vi "run.vi"(8 "error in (no error)":errorcluster, 11 "DAQ_DL090211Scaffold in":refnum<class "DAQ_DL090211Scaffold.lvclass">) -> (0 "error out":errorcluster, 3 "DAQ_DL090211Scaffold out":refnum<class "DAQ_DL090211Scaffold.lvclass">)   [LabVIEW 2010, in "DAQ_DL090211Scaffold.lvclass"]
uses:
  DAQ_DL090211Scaffold.lvclass
  internal_trigger_enum.ctl
  state_enum.ctl
  GenericDAQ/GenericDAQ/GenericDAQ.lvclass
  GenericDAQ/GenericDAQ/trigger_enum.ctl
  common/classes/ErrorController/ErrorController/class_data.vi
  common/classes/ErrorController/ErrorController/ErrorController.lvclass
panel:
  in  "Tab Control":enum32{"User", "Debug", "About"}(tab)
  out "terminate?":bool
  out "statechart loop counter":i32
  out "statechart error":errorcluster
  out "last trigger":T1
  out "loop time":u32
  # "This component has no user interface."
  # "DAQ_DL090211Scaffold\n\nImplemented by:\n- Dominik Langer, University of Zurich, Switzerland"
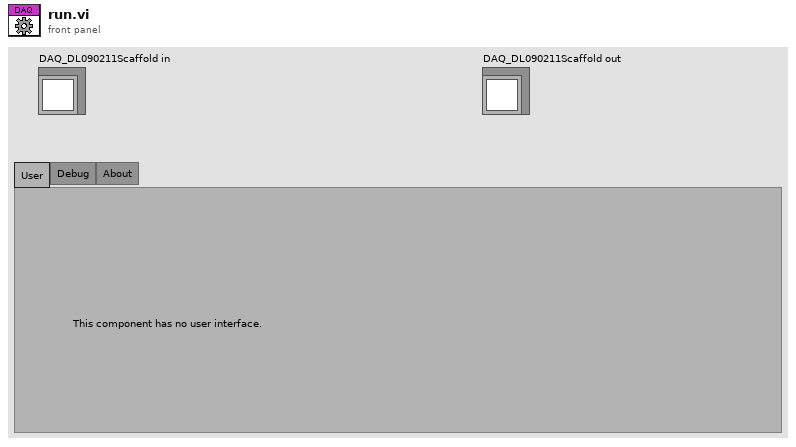
[diagram p1: front panel]
types:
  T1 = typedef "DAQ_DL090211Scaffold.lvclass/internal_trigger_enum.ctl" = enum16{"NULL", "initialise", "terminate", "start", "stop", "read", "attach observer", "detach observer", "reset"}
  T2 = typedef "DAQ_DL090211Scaffold.lvclass/state_enum.ctl" = enum16{"not acquiring", "acquiring"}
  T3 = typedef "GenericDAQ.lvclass/trigger_enum.ctl" = enum16{"NULL", "read"}
  T4 = typedef "top-level_component_type_enum.ctl" = enum16{"undefined", "ImagingMode", "ScanHead", "DAQ", "ImageAssembler", "Display", "DataCollection", "Analyser", "Stimulator", "ExperimentController", "Instrument", "Stage"}
  T5 = typedef "main_trigger_enum.ctl" = enum16{"NULL", "initialise", "terminate", "start", "stop", "change objective", "change experimentController", "change imagingMode", "save notebook", "started saving", "finished saving", "expCtr ready", "expCtr missing", "imgMd ready", "imgMd missing", "scanHd ready", "scanHd missing", "DAQ ready", "DAQ missing", "imgAsm ready", "imgAsm missing", "dataColl ready", "dataColl missing", "display ready", "display missing", "analysr ready", "analysr missing", "instrmnt ready", "instrmnt missing", "stimltr ready", "stimltr missing", "stage ready", "stage missing"}
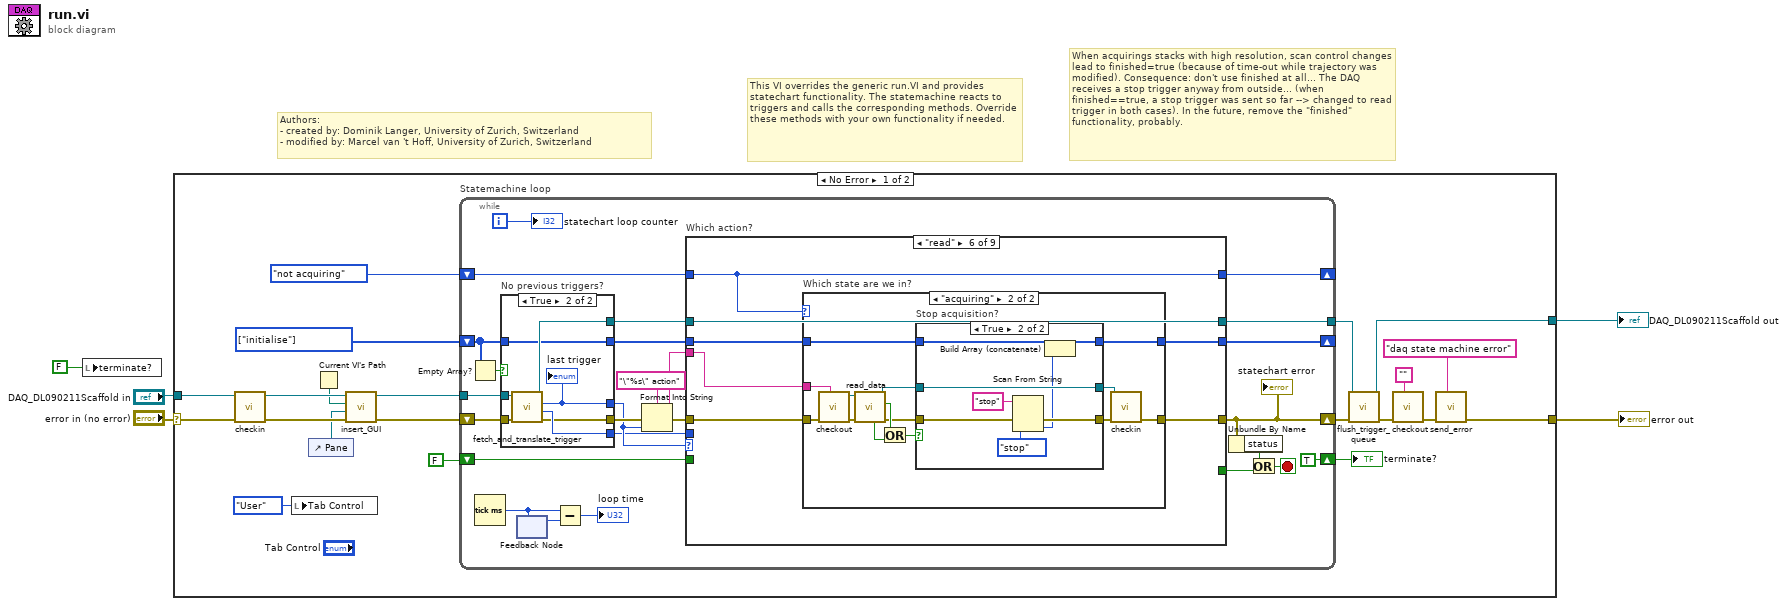
[diagram p0: block diagram]
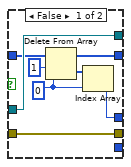
[diagram p2: hidden frame]
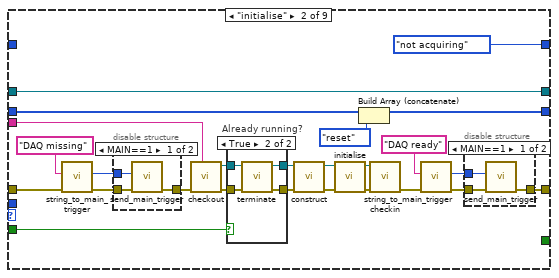
[diagram p4: hidden frame]
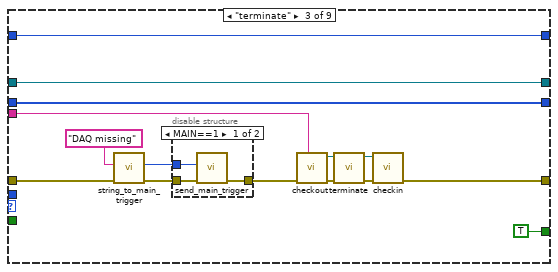
[diagram p8: hidden frame]
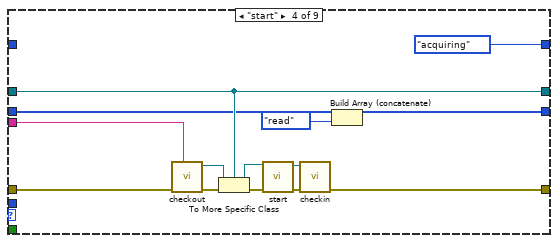
[diagram p10: hidden frame]
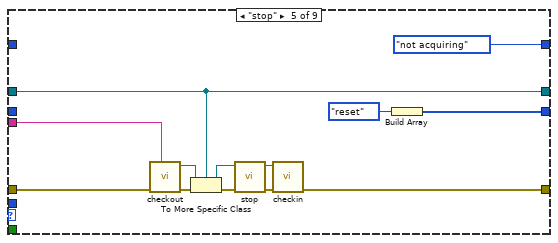
[diagram p11: hidden frame]
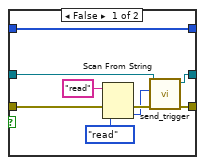
[diagram p13: hidden frame]
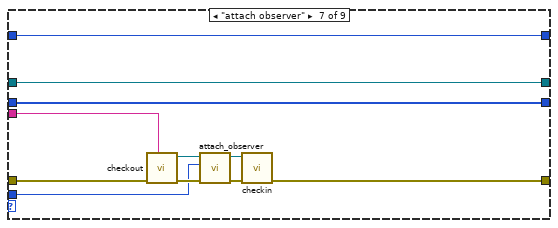
[diagram p14: hidden frame]
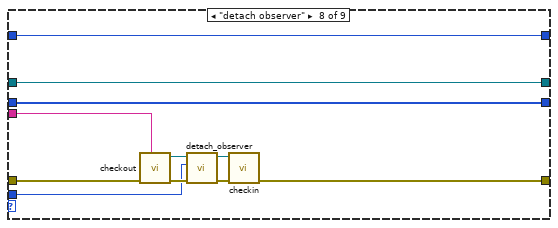
[diagram p15: hidden frame]
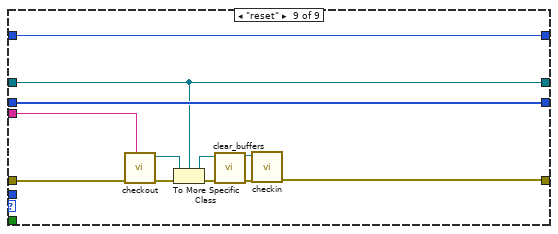
[diagram p16: hidden frame]
diagram:
  # "When acquirings stacks with high resolution, scan control changes lead to finished=true (because of time-out while trajectory was modified). Consequence: don't use finished at all... The DAQ receives a stop trigger anyway from outside... (when finished==true, a stop trigger was sent so far --> changed to read trigger in both cases). In the future, remove the \"finished\" functionality, probably."
  # "This VI overrides the generic run.VI and provides statechart functionality. The statemachine reacts to triggers and calls the corresponding methods. Override these methods with your own functionality if needed."
  # "Authors: \n- created by: Dominik Langer, University of Zurich, Switzerland\n- modified by: Marcel van 't Hoff, University of Zurich, Switzerland"
  n1 = local write "terminate?"(FALSE ("read data?")) -> ()
  n2 = case shown="No Error" "error in (no error)" {
    selector: "error in (no error)" -> [w15 w232]
    tunnel: [w6 w232] -> w4
    tunnel: [w17 w231] -> w2
    tunnel: "DAQ_DL090211Scaffold in" -> [w16 w231]
    frame No Error {
      w14 = T1[] [enum."initialise"] items=["NULL", "initialise", "terminate", "start", "stop", "read", "attach observer", "detach observer", "reset"]
      n3 = call-dynamic "checkin.vi"("error in (no error)"=w15, "GenericDAQ in"=w16) -> ("error out"=w21:errorcluster, "GenericDAQ out"=w23:refnum<class "DAQ_DL090211Scaffold.lvclass">)  [unwired: 8 in]
      n4 = local write "Tab Control"(enum32{"User", "Debug", "About"}."User" ("Tab Control")) -> ()
      n5 = control-ref of="Pane"() -> (w8:refnum<vi>)
      n6 = Current VI's Path() -> (path=w9:path)
      n7 = call-dynamic "insert_GUI.vi"("error in (no error)"=w21, "Pane"=w8, "VI path"=w9, "GenericComponent in"=w23) -> ("error out"=w7:errorcluster, "GenericComponent out"=w12:refnum<class "DAQ_DL090211Scaffold.lvclass">)  [unwired: 6 in]
      n8 = while "Statemachine loop" {
        shift-right: [TRUE] -> w11
        shift-left: FALSE -> [w45]
        shift-right: [w44] -> w20
        shift-left: w7 -> [w48]
        tunnel: w12 -> [w49]
        tunnel: [w46] -> w18
        shift-right: [w40] -> _
        shift-left: w14 -> [w39]
        shift-right: [w32] -> _
        shift-left: state_enum."not acquiring" ("state") -> [w33]
        i -> [w51]
        stop <- w50 stop-if-true
        n9 = Empty Array?(array=w39) -> (empty?=w38:bool)
        n10 = Tick Count (ms)() -> (millisecond timer value=w29:u32)
        n11 = case "No previous triggers?" shown="True" w38 {
          tunnel: w49 -> [w60 w67]
          tunnel: w48 -> [w58 w66]
          tunnel: [w60 w65] -> w47
          tunnel: [w56 w64] -> w31
          tunnel: [_ w63] -> w30
          tunnel: [w58 w62] -> w36
          tunnel: w39 -> [w59 w61]
          tunnel: [w55 w61] -> w41
          frame False {
            w53 = 0 ("index")
            n12 = Delete From Array(array=w59, length=1, index=w53) -> (deleted portion=w57:T1[], array with subset deleted=w55:T1[])
            n13 = Index Array(array=w57, index=w53) -> (element=w56:T1)
          }
          frame True {
            n14 = call-dynamic "fetch_and_translate_trigger.vi"("error in (no error)"=w66, "DAQ_DL090211Scaffold in"=w67) -> ("error out"=w62:errorcluster, "sender TLC type"=w63:T4, "trigger"=w64:T1, "DAQ_DL090211Scaffold out"=w65:refnum<class "DAQ_DL090211Scaffold.lvclass">)  [unwired: 6 in]
            "last trigger" <- w64
          }
        }
        n15 = feedback-in #1(w29) -> ()
        n16 = feedback #1() -> (w28:u32)  [unwired: 1 in]
        n17 = Subtract(x=w29, y=w28) -> (x-y=→"loop time":u32)
        n18 = Format Into String(format string="\"%s\" action", error in=w36, w31) -> (resulting string=w34:string, error out=w37:errorcluster)  [unwired: 1 in]
        n19 = case "Which action?" shown="\"read\"" w31 {
          tunnel: w47 -> [w71 w96 w125 w136 w150 w163 w207 w218 w220]
          tunnel: [w71 w96 w125 w136 w150 w163 w207 w218 w220] -> w46
          tunnel: w30 -> [_ _ _ _ _ _ w201 w212 _]
          tunnel: w37 -> [w70 w79 w114 w137 w149 w162 w202 w213 w223]
          tunnel: [w70 w76 w120 w135 w148 w161 w200 w211 w222] -> w44
          tunnel: w45 -> [_ w87 _ _ _ _ _ _ _]
          tunnel: [_ _ TRUE _ _ _ _ _ _] -> w42
          tunnel: w41 -> [w69 w85 w117 w133 _ w158 w199 w210 w230]
          tunnel: [w69 w84 w117 w132 w145 w157 w199 w210 w230] -> w40
          tunnel: w34 -> [_ w86 w116 w134 w147 w160 w198 w209 w221]
          tunnel: w33 -> [w68 _ w115 _ _ w159 w197 w208 w219]
          tunnel: [w68 state_enum."not acquiring" ("state") w115 state_enum."acquiring" ("state") state_enum."not acquiring" ("state") w159 w197 w208 w219] -> w32
          frame "NULL", Default {
          }
          frame "initialise" {
            n20 = call "string_to_main_trigger.vi"("error in (no error)"=w79, "trigger string"="DAQ missing" ("input string")) -> ("error out"=w78:errorcluster, "main trigger"=w80:T5)  [unwired: 8 in]
            n21 = disable-structure shown="MAIN==1" {
              disable-tunnel: w78 -> [w99 w100]
              disable-tunnel: [w98 w100] -> w81
              disable-tunnel: w80 -> [w97 _]
              frame condition #0 (active) {
                n22 = call "send_main_trigger.vi"("error in (no error)"=w99, "trigger"=w97) -> ("error out"=w98:errorcluster)  [unwired: 9 in]
              }
              frame condition #1 {
              }
            }
            n23 = call "checkout.vi"("locked by?"=w86, "error in (no error)"=w81) -> ("error out"=w92:errorcluster, "GenericDAQ out"=w95:refnum<class "GenericDAQ.lvclass">)  [unwired: 8 out]
            n24 = case "Already running?" shown="True" w87 {
              tunnel: w92 -> [w105 w110]
              tunnel: [w105 w109] -> w93
              tunnel: [w106 w108] -> w94
              tunnel: w95 -> [w106 w107]
              frame False {
              }
              frame True {
                n25 = call-dynamic "terminate.vi"("error in (no error)"=w110, "GenericPlugin in"=w107) -> ("error out"=w109:errorcluster, "GenericPlugin out"=w108:refnum<class "GenericDAQ.lvclass">)  [unwired: 8 out]
              }
            }
            n26 = call-dynamic "construct.vi"("error in (no error)"=w93, "GenericPlugin in"=w94) -> ("error out"=w89:errorcluster, "GenericPlugin out"=w90:refnum<class "GenericDAQ.lvclass">)  [unwired: 2 in, 6 out]
            n27 = call-dynamic "initialise.vi"("error in (no error)"=w89, "GenericPlugin in"=w90) -> ("error out"=w91:errorcluster, "GenericPlugin out"=w88:refnum<class "GenericDAQ.lvclass">)  [unwired: 8 out]
            n28 = Build Array (concatenate)(w85, internal_trigger_enum."reset" ("last trigger 2")) -> (w84:T1[])
            n29 = call-dynamic "checkin.vi"("error in (no error)"=w91, "GenericDAQ in"=w88) -> ("error out"=w75:errorcluster)  [unwired: 8 in, 1 out]
            n30 = call "string_to_main_trigger.vi"("error in (no error)"=w75, "trigger string"="DAQ ready" ("input string")) -> ("error out"=w74:errorcluster, "main trigger"=w72:T5)  [unwired: 8 in]
            n31 = disable-structure shown="MAIN==1" {
              disable-tunnel: w74 -> [w103 w104]
              disable-tunnel: [w102 w104] -> w76
              disable-tunnel: w72 -> [w101 _]
              frame condition #0 (active) {
                n32 = call "send_main_trigger.vi"("error in (no error)"=w103, "trigger"=w101) -> ("error out"=w102:errorcluster)  [unwired: 9 in]
              }
              frame condition #1 {
              }
            }
          }
          frame "terminate" {
            n33 = call "string_to_main_trigger.vi"("error in (no error)"=w114, "trigger string"="DAQ missing" ("input string")) -> ("error out"=w113:errorcluster, "main trigger"=w111:T5)  [unwired: 8 in]
            n34 = disable-structure shown="MAIN==1" {
              disable-tunnel: w113 -> [w128 w129]
              disable-tunnel: [w127 w129] -> w118
              disable-tunnel: w111 -> [w126 _]
              frame condition #0 (active) {
                n35 = call "send_main_trigger.vi"("error in (no error)"=w128, "trigger"=w126) -> ("error out"=w127:errorcluster)  [unwired: 9 in]
              }
              frame condition #1 {
              }
            }
            n36 = call "checkout.vi"("locked by?"=w116, "error in (no error)"=w118) -> ("error out"=w124:errorcluster, "GenericDAQ out"=w123:refnum<class "GenericDAQ.lvclass">)  [unwired: 8 out]
            n37 = call-dynamic "terminate.vi"("error in (no error)"=w124, "GenericPlugin in"=w123) -> ("error out"=w122:errorcluster, "GenericPlugin out"=w121:refnum<class "GenericDAQ.lvclass">)  [unwired: 8 out]
            n38 = call-dynamic "checkin.vi"("error in (no error)"=w122, "GenericDAQ in"=w121) -> ("error out"=w120:errorcluster)  [unwired: 8 in, 1 out]
          }
          frame "start" {
            n39 = call "checkout.vi"("locked by?"=w134, "error in (no error)"=w137) -> ("error out"=w143:errorcluster, "GenericDAQ out"=w142:refnum<class "GenericDAQ.lvclass">)  [unwired: 8 out]
            n40 = To More Specific Class(target class=w136, reference=w142, error in=w143) -> (specific class reference=w140:refnum<class "DAQ_DL090211Scaffold.lvclass">, error out=w141:errorcluster)
            n41 = call-dynamic "start.vi"("error in (no error)"=w141, "DL090211DAQScaffold in"=w140) -> ("error out"=w139:errorcluster, "DL090211DAQScaffold out"=w138:refnum<class "DAQ_DL090211Scaffold.lvclass">)  [unwired: 8 out]
            n42 = call-dynamic "checkin.vi"("error in (no error)"=w139, "GenericDAQ in"=w138) -> ("error out"=w135:errorcluster)  [unwired: 8 in, 1 out]
            n43 = Build Array (concatenate)(w133, internal_trigger_enum."read" ("last trigger 2")) -> (w132:T1[])
          }
          frame "stop" {
            n44 = call "checkout.vi"("locked by?"=w147, "error in (no error)"=w149) -> ("error out"=w156:errorcluster, "GenericDAQ out"=w155:refnum<class "GenericDAQ.lvclass">)  [unwired: 8 out]
            n45 = To More Specific Class(target class=w150, reference=w155, error in=w156) -> (specific class reference=w153:refnum<class "DAQ_DL090211Scaffold.lvclass">, error out=w154:errorcluster)
            n46 = call-dynamic "stop.vi"("error in (no error)"=w154, "DAQ_DL090211Scaffold in"=w153) -> ("error out"=w152:errorcluster, "DAQ_DL090211Scaffold out"=w151:refnum<class "DAQ_DL090211Scaffold.lvclass">)  [unwired: 8 in]
            n47 = call-dynamic "checkin.vi"("error in (no error)"=w152, "GenericDAQ in"=w151) -> ("error out"=w148:errorcluster)  [unwired: 8 in, 1 out]
            n48 = Build Array(internal_trigger_enum."reset" ("last trigger 2")) -> (w145:T1[])
          }
          frame "read" {
            n49 = case "Which state are we in?" shown="\"acquiring\"" w159 {
              tunnel: w162 -> [w165 w179]
              tunnel: [w165 w172] -> w161
              tunnel: w160 -> [_ w169]
              tunnel: w158 -> [w164 w167]
              tunnel: [w164 w166] -> w157
              frame "not acquiring", Default {
              }
              frame "acquiring" {
                n50 = call "checkout.vi"("locked by?"=w169, "error in (no error)"=w179) -> ("error out"=w177:errorcluster, "GenericDAQ out"=w178:refnum<class "GenericDAQ.lvclass">)  [unwired: 8 in]
                n51 = call-dynamic "read_data.vi"("error in (no error)"=w177, "GenericDAQ in"=w178) -> ("error out"=w170:errorcluster, "finished?"=w175:bool, "GenericDAQ out"=w176:refnum<class "GenericDAQ.lvclass">, "buffer overflow?"=w174:bool)  [unwired: 6 out]
                n52 = Or(x=w175, y=w174) -> (x .or. y?=w168:bool)
                n53 = case "Stop acquisition?" shown="True" w168 {
                  tunnel: w176 -> [w188 w196]
                  tunnel: [w187 w193] -> w173
                  tunnel: [w186 w196] -> w171
                  tunnel: w170 -> [w184 w194]
                  tunnel: w167 -> [w180 w195]
                  tunnel: [w180 w191] -> w166
                  frame False {
                    n54 = Scan From String(input string="read", error in=w184, default 1=trigger_enum."read" ("message")) -> (error out=w183:errorcluster, output 1=w182:T3)  [unwired: 2 in, 2 out]
                    n55 = call-dynamic "send_trigger.vi"("error in (no error)"=w183, "message"=w182, "GenericDAQ in"=w188) -> ("error out"=w187:errorcluster, "GenericDAQ out"=w186:refnum<class "GenericDAQ.lvclass">)  [unwired: 7 in]
                  }
                  frame True {
                    n56 = Scan From String(input string="stop", error in=w194, default 1=internal_trigger_enum."stop" ("last trigger 2")) -> (error out=w193:errorcluster, output 1=w190:T1)  [unwired: 2 in, 2 out]
                    n57 = Build Array (concatenate)(w195, w190) -> (w191:T1[])
                  }
                }
                n58 = call-dynamic "checkin.vi"("error in (no error)"=w173, "GenericDAQ in"=w171) -> ("error out"=w172:errorcluster)  [unwired: 8 in, 1 out]
              }
            }
          }
          frame "attach observer" {
            n59 = call "checkout.vi"("locked by?"=w198, "error in (no error)"=w202) -> ("error out"=w206:errorcluster, "GenericDAQ out"=w205:refnum<class "GenericDAQ.lvclass">)  [unwired: 8 in]
            n60 = call-dynamic "attach_observer.vi"("error in (no error)"=w206, "top-level component type"=w201, "GenericToplevelComponent in"=w205) -> ("error out"=w204:errorcluster, "GenericToplevelComponent out"=w203:refnum<class "GenericDAQ.lvclass">)  [unwired: 7 in]
            n61 = call-dynamic "checkin.vi"("error in (no error)"=w204, "GenericDAQ in"=w203) -> ("error out"=w200:errorcluster)  [unwired: 8 in, 1 out]
          }
          frame "detach observer" {
            n62 = call "checkout.vi"("locked by?"=w209, "error in (no error)"=w213) -> ("error out"=w217:errorcluster, "GenericDAQ out"=w216:refnum<class "GenericDAQ.lvclass">)  [unwired: 8 in]
            n63 = call-dynamic "detach_observer.vi"("error in (no error)"=w217, "top-level component type"=w212, "GenericToplevelComponent in"=w216) -> ("error out"=w215:errorcluster, "GenericToplevelComponent out"=w214:refnum<class "GenericDAQ.lvclass">)  [unwired: 7 in]
            n64 = call-dynamic "checkin.vi"("error in (no error)"=w215, "GenericDAQ in"=w214) -> ("error out"=w211:errorcluster)  [unwired: 8 in, 1 out]
          }
          frame "reset" {
            n65 = call "checkout.vi"("locked by?"=w221, "error in (no error)"=w223) -> ("error out"=w229:errorcluster, "GenericDAQ out"=w228:refnum<class "GenericDAQ.lvclass">)  [unwired: 8 out]
            n66 = To More Specific Class(target class=w220, reference=w228, error in=w229) -> (specific class reference=w226:refnum<class "DAQ_DL090211Scaffold.lvclass">, error out=w227:errorcluster)
            n67 = call-dynamic "clear_buffers.vi"("error in (no error)"=w227, "GenericDAQ in"=w226) -> ("error out"=w225:errorcluster, "GenericDAQ out"=w224:refnum<class "DAQ_DL090211Scaffold.lvclass">)  [unwired: 8 out]
            n68 = call-dynamic "checkin.vi"("error in (no error)"=w225, "GenericDAQ in"=w224) -> ("error out"=w222:errorcluster)  [unwired: 8 in, 1 out]
          }
        }
        "statechart error" <- w44
        n69 = Unbundle By Name(w44) -> ("status"=w43:bool)
        n70 = Or(x=w43, y=w42) -> (x .or. y?=w50:bool)
        "statechart loop counter" <- w51
      }
      "terminate?" <- w11
      n71 = call-dynamic "flush_trigger_queue.vi"("error in (no error)"=w20, "GenericToplevelComponent in"=w18) -> ("error out"=w19:errorcluster, "GenericToplevelComponent out"=w17:refnum<class "DAQ_DL090211Scaffold.lvclass">)  [unwired: 8 in]
      n72 = call "checkout.vi"("locked by?"="", "error in (no error)"=w19) -> ("error out"=w22:errorcluster)  [unwired: 9 out]
      n73 = call "send_error.vi"("additional message"="daq state machine error", "error in (no error)"=w22) -> ("error out"=w6:errorcluster)  [unwired: 9 in]
    }
    frame Error {
    }
  }
  "error out" <- w4
  "DAQ_DL090211Scaffold out" <- w2
